vi "Set Created Events.vi"(10 "Created Events":map{string, refnum<data-value>}(c390), 11 "Addresses in":refnum<class "Addresses.lvclass">) -> (3 "Addresses out":refnum<class "Addresses.lvclass">)   [LabVIEW 2021, in "jettl.lvlib" / "Addresses.lvlib" / "Addresses.lvclass"]
uses:
  Addresses.lvclass
  Msg Strategy/Msg Strategy.lvclass
  Addresses.lvclass/Addresses.ctl
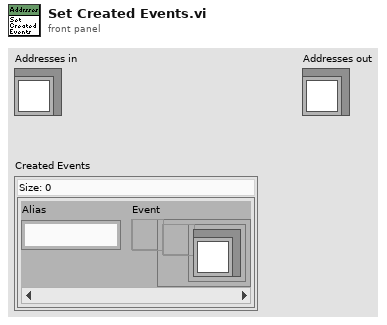
[diagram p1: front panel]
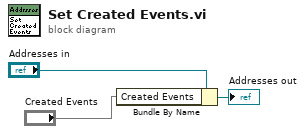
[diagram p0: block diagram]
diagram:
  n1 = Bundle By Name(cluster="Addresses in", "Created Events"="Created Events") -> (→"Addresses out":refnum<class "Addresses.lvclass">)
